vi "HEWH Data File Info String.vi"(9 "Set PointOut":u8=140, 10 "GEA2 Set Mode":T1=enum."HighDemand") -> (2 "Info string":string)   [LabVIEW 2014]
uses:
  Utility/GEA2 Commands/HEWH/Type Definitions/HEWH_Mode.ctl
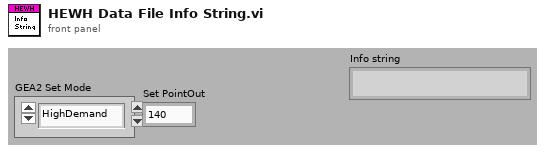
[diagram p1: front panel]
types:
  T1 = typedef "HEWH_Mode.ctl" = enum16{"Hybrid", "Std Electric", "eHeat", "HighDemand", "Vacation"}
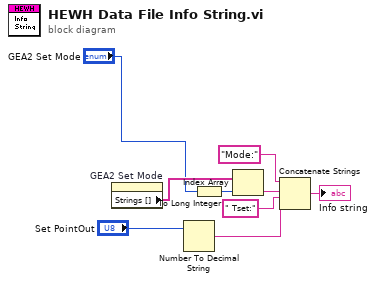
[diagram p0: block diagram]
diagram:
  n1 = property on="GEA2 Set Mode" class="Enum (strict)"() -> ("Strings []"=w4:string[])  [unwired: 2 in, 2 out]
  n2 = Number To Decimal String(number="Set PointOut") -> (decimal integer string=w6:string)  [unwired: 1 in]
  n3 = To Long Integer(number="GEA2 Set Mode") -> (32bit integer=w5:i32)
  n4 = Index Array(array=w4, index=w5) -> (element=w8:string)
  n5 = Concatenate Strings("Mode:" ("Test_Type In:"), w8, " Tset:" ("Test_Type In:"), w6) -> (→"Info string":string)
